vi "shutter_temp.vi"(7 "converter box version":i16=1 min=1 max=2, 11 "open?":bool) -> ()   [LabVIEW 2010]
uses:
  <vilib>/eio/EIONode/EIONode.xnode
  <vilib>/rvi/eio/nirviEIOImplementation/nirviEIOImplementation.xnode
  <vilib>/rvi/eio/common/nirviEmuClasses.ctl
  <vilib>/rvi/eio/common/nirviEmuTemplateMethod_noerrors.vi
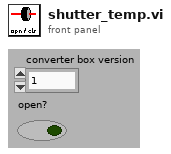
[diagram p1: front panel]
types:
  T1 = typedef "nirviEmuClasses.ctl" = enum16{"IO Read", "IO Write", "Method", "Property Read", "Property Write"}
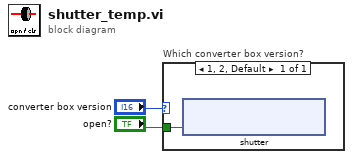
[diagram p0: block diagram]
diagram:
  n1 = case "Which converter box version?" shown="1, 2, Default" "converter box version" {
    tunnel: "open?" -> [w3]
    frame 1, 2, Default {
      n2 = xnode "shutter"("Connector2/DIO32"=w3) -> ()  [unwired: 1 in, 1 out]
    }
  }
